vi "DecodePrivateKey.vi"(3 "error in (no error) 2":errorcluster, 4 "Private Key":string) -> (0 "error out":errorcluster, 1 "d":cluster{"P/N":bool, "Array":u64[]}, 2 "n":cluster{"P/N":bool, "Array":u64[]})   [LabVIEW 2023]
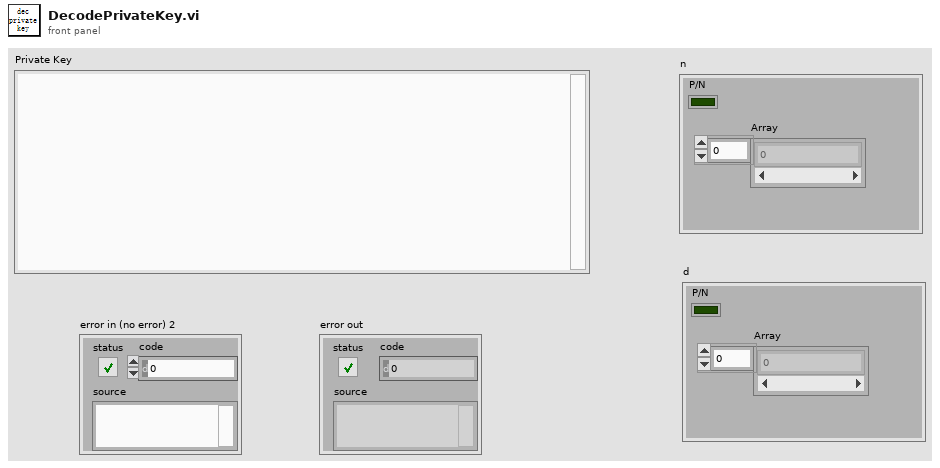
[diagram p1: front panel]
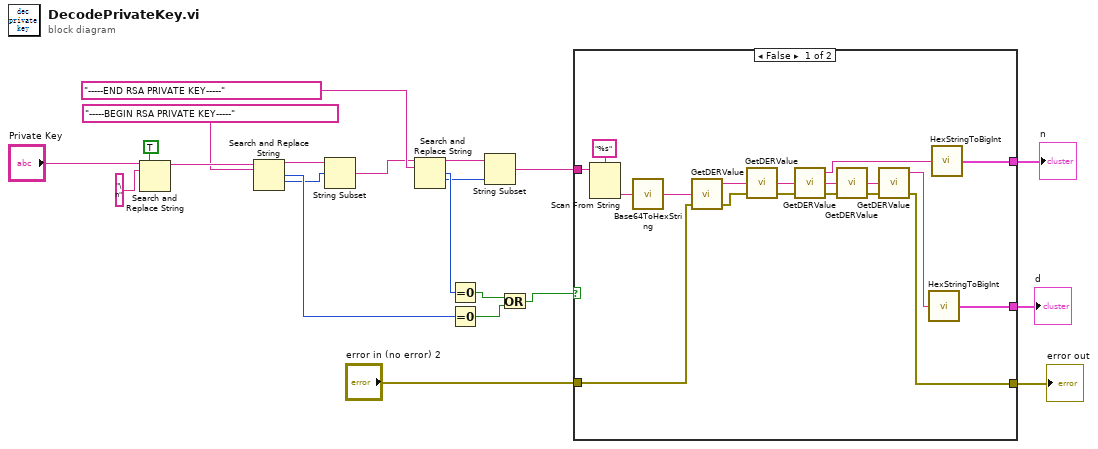
[diagram p0: block diagram]
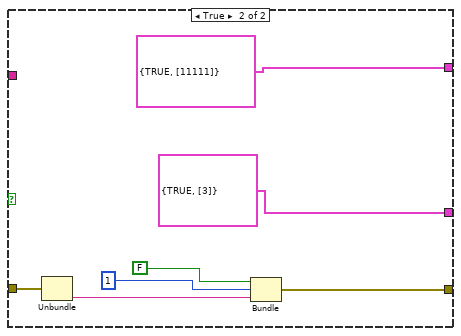
[diagram p2: hidden frame]
diagram:
  n1 = Search and Replace String(replace all?=TRUE, input string="Private Key", search string="\n") -> (result string=w18:string)  [unwired: 5 in, 3 out]
  n2 = Search and Replace String(input string=w18, search string="-----BEGIN RSA PRIVATE KEY-----") -> (result string=w13:string, number of replacements=w15:i32, offset past replacement=w12:i32)  [unwired: 6 in, 1 out]
  n3 = String Subset(string=w13, offset (0)=w12) -> (substring=w11:string)  [unwired: 1 in]
  n4 = Search and Replace String(input string=w11, search string="-----END RSA PRIVATE KEY-----") -> (result string=w10:string, number of replacements=w14:i32, offset past replacement=w9:i32)  [unwired: 6 in, 1 out]
  n5 = Equal To 0?(x=w14) -> (x = 0?=w7:bool)
  n6 = Equal To 0?(x=w15) -> (x = 0?=w6:bool)
  n7 = String Subset(string=w10, length (rest)=w9) -> (substring=w8:string)  [unwired: 1 in]
  n8 = Or(x=w7, y=w6) -> (x .or. y?=w5:bool)
  n9 = case shown="False" w5 {
    tunnel: w8 -> [w38 _]
    tunnel: [w33 cluster{bool, u64[]} {TRUE, [11111]}] -> w4
    tunnel: [w32 cluster{bool, u64[]} {TRUE, [3]}] -> w3
    tunnel: [w22 w40] -> w2
    tunnel: "error in (no error) 2" -> [w29 w44]
    frame False {
      n10 = Scan From String(format string="%s", input string=w38) -> (output 1=w37:string)  [unwired: 3 in, 3 out]
      n11 = call "Base64ToHexString.vi"("BASE64 string"=w37) -> ("Hex"=w35:string)
      n12 = call "GetDERValue.vi"("error in (no error)"=w29, "DER"=w35) -> ("error out"=w31:errorcluster, "value"=w34:string)  [unwired: 1 in, 1 out]
      n13 = call "GetDERValue.vi"("error in (no error)"=w31, "DER"=w34) -> ("error out"=w30:errorcluster, "remaining"=w36:string)  [unwired: 1 in, 1 out]
      n14 = call "GetDERValue.vi"("error in (no error)"=w30, "DER"=w36) -> ("error out"=w26:errorcluster, "remaining"=w28:string, "value"=w24:string)  [unwired: 1 in]
      n15 = call "GetDERValue.vi"("error in (no error)"=w26, "DER"=w28) -> ("error out"=w25:errorcluster, "remaining"=w27:string)  [unwired: 1 in, 1 out]
      n16 = call "GetDERValue.vi"("error in (no error)"=w25, "DER"=w27) -> ("error out"=w22:errorcluster, "value"=w23:string)  [unwired: 1 in, 1 out]
      n17 = call "HexStringToBigInt.vi"("String (hex)"=w23) -> ("Int"=w32:cluster{"P/N":bool, "Array":u64[]})
      n18 = call "HexStringToBigInt.vi"("String (hex)"=w24) -> ("Int"=w33:cluster{"P/N":bool, "Array":u64[]})
    }
    frame True {
      n19 = Unbundle(w44) -> ("source"=w43:string)  [unwired: 2 out]
      n20 = Bundle(FALSE, 1, "source"=w43) -> (w40:cluster{bool, i32, "source":string})  [unwired: 1 in]
    }
  }
  "n" <- w4
  "d" <- w3
  "error out" <- w2
